vi "SMC HECR.vi"() -> ()   [LabVIEW 2015]
doc: "Example VI that demonstrates all library features."
uses:
  PL SMC HECR.lvclass
panel:
  out "state":T1
  in  "configuration":T2={"control mode"=0, "Ttarget, °C"=25.0, "offset, °C"=0.0, "PID"={"PB range, °C"=6.0, "integral time, s"=18.0, "differential time, s"=0.0}, "heat output limit, %"=100.0, "cool output limit, %"=-100.0} {"control mode" items=["stop", "normal", "auto tuning", "learning", "external tune"]}
  in  "parity":enum16{"None", "Odd", "Even"}(ring)
  in  "data bits":u16(ring)=8 items=["7"=7, "8"=8]
  in  "baud rate":u32(ring)=1200 items=["600"=600, "1200"=1200, "2400"=2400, "4800"=4800, "9600"=9600, "19200"=19200]
  in  "stop bits":u16(ring)=10 items=["1.0"=10, "2.0"=20]
  in  "address":u8=1
  in  "port":refnum<visa-resource-name>
  out "HECR":refnum<class "PL SMC HECR.lvclass">
  out "error":errorcluster
  in  "stop":bool
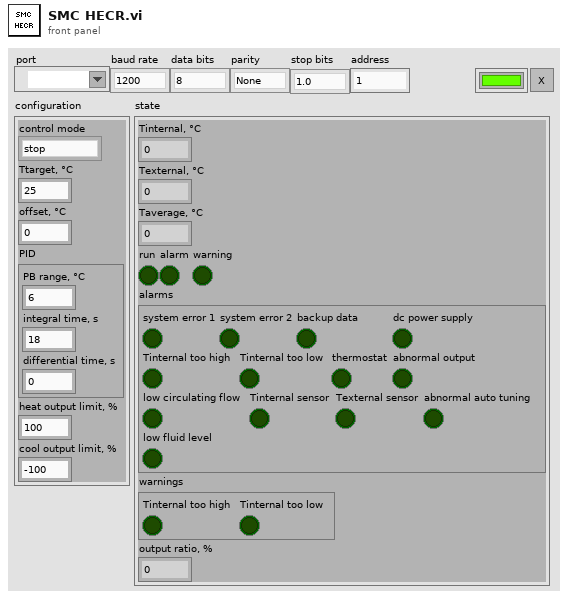
[diagram p1: front panel]
types:
  T1 = cluster{"Tinternal, °C":dbl, "Texternal, °C":dbl, "Taverage, °C":dbl, "run":bool, "alarm":bool, "warning":bool, "alarms":cluster{"system error 1":bool, "system error 2":bool, "backup data":bool, "dc power supply":bool, "Tinternal too high":bool, "Tinternal too low":bool, "thermostat":bool, "abnormal output":bool, "low circulating flow":bool, "Tinternal sensor":bool, "Texternal sensor":bool, "abnormal auto tuning":bool, "low fluid level":bool}, "warnings":cluster{"Tinternal too high":bool, "Tinternal too low":bool}, "output ratio, %":dbl}
  T2 = cluster{"control mode":u16, "Ttarget, °C":dbl, "offset, °C":dbl, "PID":cluster{"PB range, °C":dbl, "integral time, s":dbl, "differential time, s":dbl}, "heat output limit, %":dbl, "cool output limit, %":dbl}
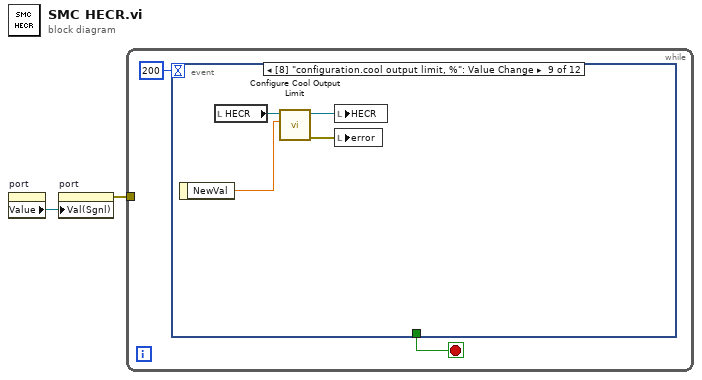
[diagram p0: block diagram]
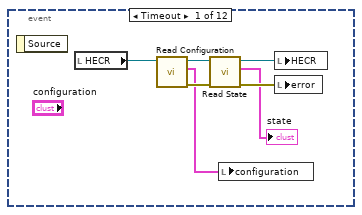
[diagram p2: hidden frame]
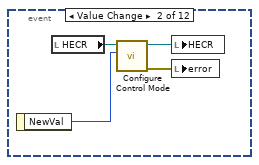
[diagram p3: hidden frame]
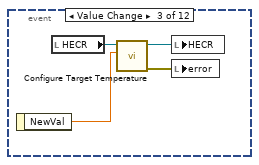
[diagram p4: hidden frame]
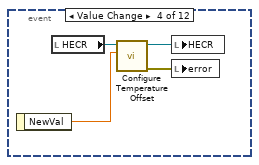
[diagram p5: hidden frame]
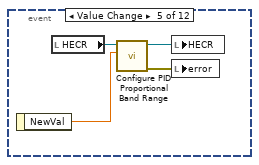
[diagram p6: hidden frame]
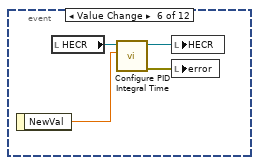
[diagram p7: hidden frame]
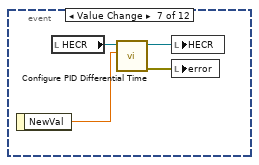
[diagram p8: hidden frame]
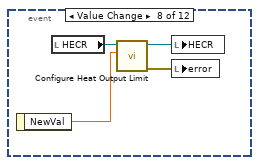
[diagram p9: hidden frame]
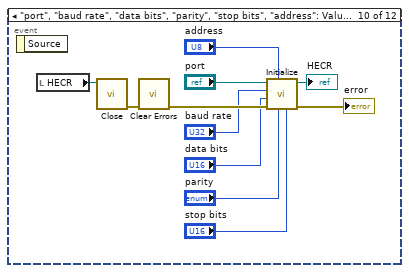
[diagram p10: hidden frame]
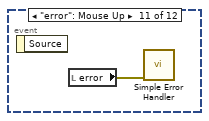
[diagram p11: hidden frame]
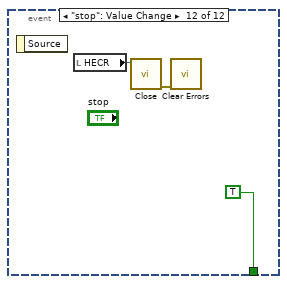
[diagram p12: hidden frame]
diagram:
  n1 = property on="port" class="VISAName"() -> ("Value"=w1:refnum<visa-resource-name>)  [unwired: 2 in, 2 out]
  n2 = property on="port" class="VISAName"("Val(Sgnl)"=w1) -> (error out=w2:errorcluster)  [unwired: 2 in, 1 out]
  n3 = while {
    tunnel: w2 -> [_]
    stop <- w3 stop-if-true
    n4 = event shown="[8] \"configuration.cool output limit, %\": Value Change" {
      selector: _ -> [_ _ _ _ _ _ _ _ _ _ _ _]
      dyn-events: _ -> [_ _ _ _ _ _ _ _ _ _ _ _]
      timeout: 200 -> [_ _ _ _ _ _ _ _ _ _ _ _]
      tunnel: [_ _ _ _ _ _ _ _ _ _ _ TRUE ("stop")] -> w3
      event Timeout {
        n5 = event-data() -> ()  [unwired: 1 in, 1 out]
        n6 = local read "HECR"() -> (w11:refnum<class "PL SMC HECR.lvclass">)
        n7 = call "Read Configuration.vi"("HECR in"=w11) -> ("error out"=w7:errorcluster, "configuration"=w6:T2, "HECR out"=w10:refnum<class "PL SMC HECR.lvclass">)  [unwired: 8 in]
        n8 = call "Read State.vi"("error in (no error)"=w7, "HECR in"=w10) -> ("error out"=w8:errorcluster, "state"=→"state":T1, "HECR out"=w9:refnum<class "PL SMC HECR.lvclass">)  [unwired: 7 in]
        n9 = local write "configuration"(w6) -> ()
        n10 = local write "HECR"(w9) -> ()
        n11 = local write "error"(w8) -> ()
      }
      event "configuration.control mode": Value Change {
        n12 = event-data() -> ("NewVal"=w12:u16)  [unwired: 1 in]
        n13 = local read "HECR"() -> (w15:refnum<class "PL SMC HECR.lvclass">)
        n14 = call "Configure Control Mode.vi"("control mode"=w12, "HECR in"=w15) -> ("error out"=w13:errorcluster, "HECR out"=w14:refnum<class "PL SMC HECR.lvclass">)  [unwired: 8 in]
        n15 = local write "HECR"(w14) -> ()
        n16 = local write "error"(w13) -> ()
      }
      event "configuration.Ttarget, °C": Value Change {
        n17 = event-data() -> ("NewVal"=w16:dbl)  [unwired: 1 in]
        n18 = local read "HECR"() -> (w19:refnum<class "PL SMC HECR.lvclass">)
        n19 = call "Configure Target Temperature.vi"("Ttarget, °C"=w16, "HECR in"=w19) -> ("error out"=w17:errorcluster, "HECR out"=w18:refnum<class "PL SMC HECR.lvclass">)  [unwired: 8 in]
        n20 = local write "HECR"(w18) -> ()
        n21 = local write "error"(w17) -> ()
      }
      event "configuration.offset, °C": Value Change {
        n22 = event-data() -> ("NewVal"=w20:dbl)  [unwired: 1 in]
        n23 = local read "HECR"() -> (w23:refnum<class "PL SMC HECR.lvclass">)
        n24 = call "Configure Temperature Offset.vi"("offset, °C"=w20, "HECR in"=w23) -> ("error out"=w21:errorcluster, "HECR out"=w22:refnum<class "PL SMC HECR.lvclass">)  [unwired: 8 in]
        n25 = local write "HECR"(w22) -> ()
        n26 = local write "error"(w21) -> ()
      }
      event "configuration.PID.PB range, °C": Value Change {
        n27 = event-data() -> ("NewVal"=w24:dbl)  [unwired: 1 in]
        n28 = local read "HECR"() -> (w27:refnum<class "PL SMC HECR.lvclass">)
        n29 = call "Configure PID Proportional Band Range.vi"("PB range, °C"=w24, "HECR in"=w27) -> ("error out"=w25:errorcluster, "HECR out"=w26:refnum<class "PL SMC HECR.lvclass">)  [unwired: 8 in]
        n30 = local write "HECR"(w26) -> ()
        n31 = local write "error"(w25) -> ()
      }
      event "configuration.PID.integral time, s": Value Change {
        n32 = event-data() -> ("NewVal"=w28:dbl)  [unwired: 1 in]
        n33 = local read "HECR"() -> (w31:refnum<class "PL SMC HECR.lvclass">)
        n34 = call "Configure PID Integral Time.vi"("integral time, s"=w28, "HECR in"=w31) -> ("error out"=w29:errorcluster, "HECR out"=w30:refnum<class "PL SMC HECR.lvclass">)  [unwired: 8 in]
        n35 = local write "HECR"(w30) -> ()
        n36 = local write "error"(w29) -> ()
      }
      event "configuration.PID.differential time, s": Value Change {
        n37 = event-data() -> ("NewVal"=w32:dbl)  [unwired: 1 in]
        n38 = local read "HECR"() -> (w35:refnum<class "PL SMC HECR.lvclass">)
        n39 = call "Configure PID Differential Time.vi"("differential time, s"=w32, "HECR in"=w35) -> ("error out"=w33:errorcluster, "HECR out"=w34:refnum<class "PL SMC HECR.lvclass">)  [unwired: 8 in]
        n40 = local write "HECR"(w34) -> ()
        n41 = local write "error"(w33) -> ()
      }
      event "configuration.heat output limit, %": Value Change {
        n42 = event-data() -> ("NewVal"=w36:dbl)  [unwired: 1 in]
        n43 = local read "HECR"() -> (w39:refnum<class "PL SMC HECR.lvclass">)
        n44 = call "Configure Heat Output Limit.vi"("heat output limit, %"=w36, "HECR in"=w39) -> ("error out"=w37:errorcluster, "HECR out"=w38:refnum<class "PL SMC HECR.lvclass">)  [unwired: 8 in]
        n45 = local write "HECR"(w38) -> ()
        n46 = local write "error"(w37) -> ()
      }
      event "configuration.cool output limit, %": Value Change {
        n47 = event-data() -> ("NewVal"=w40:dbl)  [unwired: 1 in]
        n48 = local read "HECR"() -> (w43:refnum<class "PL SMC HECR.lvclass">)
        n49 = call "Configure Cool Output Limit.vi"("cool output limit, %"=w40, "HECR in"=w43) -> ("error out"=w41:errorcluster, "HECR out"=w42:refnum<class "PL SMC HECR.lvclass">)  [unwired: 8 in]
        n50 = local write "HECR"(w42) -> ()
        n51 = local write "error"(w41) -> ()
      }
      event "port", "baud rate", "data bits", "parity", "stop bits", "address": Value Change {
        n52 = event-data() -> ()  [unwired: 1 in, 1 out]
        n53 = local read "HECR"() -> (w52:refnum<class "PL SMC HECR.lvclass">)
        n54 = call-dynamic "Close.vi"("HECR in"=w52) -> ("error out"=w51:errorcluster)  [unwired: 10 in]
        n55 = call <vilib>:"Clear Errors.vi"("error in (no error)"=w51) -> ("error out"=w50:errorcluster)  [unwired: 5 in, 1 out]
        n56 = call "Initialize.vi"("stop bits (1.0)"="stop bits", "parity (none)"="parity", "address (1)"="address", "error in (no error)"=w50, "data bits (8)"="data bits", "baud rate (1200)"="baud rate", "port"="port") -> ("error out"=→"error":errorcluster, "HECR out"=→"HECR":refnum<class "PL SMC HECR.lvclass">)  [unwired: 3 in]
      }
      event "error": Mouse Up {
        n57 = event-data() -> ()  [unwired: 1 in, 1 out]
        n58 = local read "error"() -> (w55:errorcluster)
        n59 = call <vilib>:"Simple Error Handler.vi"("error in (no error)"=w55) -> ()  [unwired: 4 in, 5 out]
      }
      event "stop": Value Change {
        n60 = event-data() -> ()  [unwired: 1 in, 1 out]
        n61 = local read "HECR"() -> (w58:refnum<class "PL SMC HECR.lvclass">)
        n62 = call-dynamic "Close.vi"("HECR in"=w58) -> ("error out"=w56:errorcluster)  [unwired: 10 in]
        n63 = call <vilib>:"Clear Errors.vi"("error in (no error)"=w56) -> ()  [unwired: 5 in, 2 out]
      }
    }
  }
